vi "Delete Temp Files.vi"(8 "error in (no error)":errorcluster) -> (0 "error out":errorcluster)   [LabVIEW 2017]
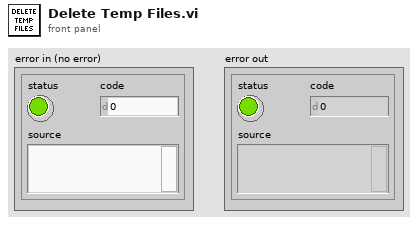
[diagram p1: front panel]
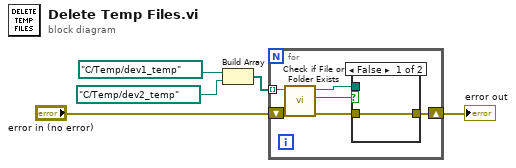
[diagram p0: block diagram]
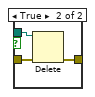
[diagram p2: hidden frame]
diagram:
  n1 = Build Array(path "C:/Temp/dev1_temp" ("file path (dialog if empty)"), path "C:/Temp/dev2_temp" ("file path (dialog if empty)")) -> (w5:path[])
  n2 = for {
    shift-right: [w8] -> w1
    shift-left: "error in (no error)" -> [w7]
    tunnel: w5 -> [w6] mode=indexing
    n3 = call <vilib>:"Check if File or Folder Exists.vi"("error in (no error)"=w7, "path"=w6) -> ("error out"=w9:errorcluster, "file or folder exists?"=w11:bool, "dup path"=w10:path)  [unwired: 7 in]
    n4 = case shown="False" w11 {
      tunnel: w10 -> [_ w15]
      tunnel: w9 -> [w12 w14]
      tunnel: [w12 w13] -> w8
      frame False {
      }
      frame True {
        n5 = Delete(path (use dialog)=w15, error in=w14) -> (error out=w13:errorcluster)  [unwired: 3 in, 2 out]
      }
    }
  }
  "error out" <- w1
